vi "FindRequestByType.vi"(8 "ErrorIn":errorcluster={"status"=TRUE, "code"=6, "source"="Device disconnected"}, 11 "RequestType":T2=enum."Reset") -> (0 "ErrorOut":errorcluster={"status"=TRUE, "code"=6, "source"="Device disconnected"}, 3 "Request":T1={"Type"=enum."Reset", "Command"="", "Mode"={"Direction"=enum."TransmitOnly", "BytesToRead"=0}} {"Mode"."BytesToRead" min=1 max=4000000000 step=1})   [LabVIEW 2016]
doc: "Find Request cluster using its type. If the is no match during comparison with AvailableRequests, VI throws an error."
uses:
  RequestType.ctl
  Request.ctl
  FTDI/COMMode.ctl
  FTDI/COMDirection.ctl
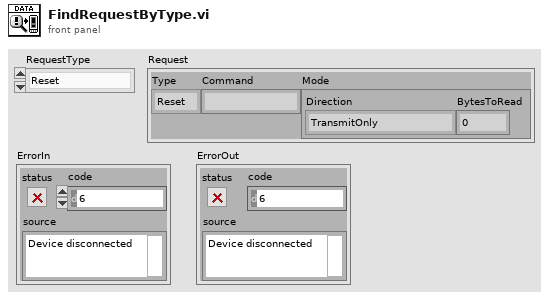
[diagram p1: front panel]
types:
  T1 = typedef "Request.ctl" = cluster{"Type":T2, "Command":string, "Mode":T3}
  T2 = typedef "RequestType.ctl" = enum16{"NONE", "Reset", "Hello", "GetPacketsNr", "GetMeasFreq", "GetPacket"}
  T3 = typedef "COMMode.ctl" = cluster{"Direction":T4, "BytesToRead":u32}
  T4 = typedef "COMDirection.ctl" = enum16{"CommandAndResponse", "ReceiveOnly", "TransmitOnly"}
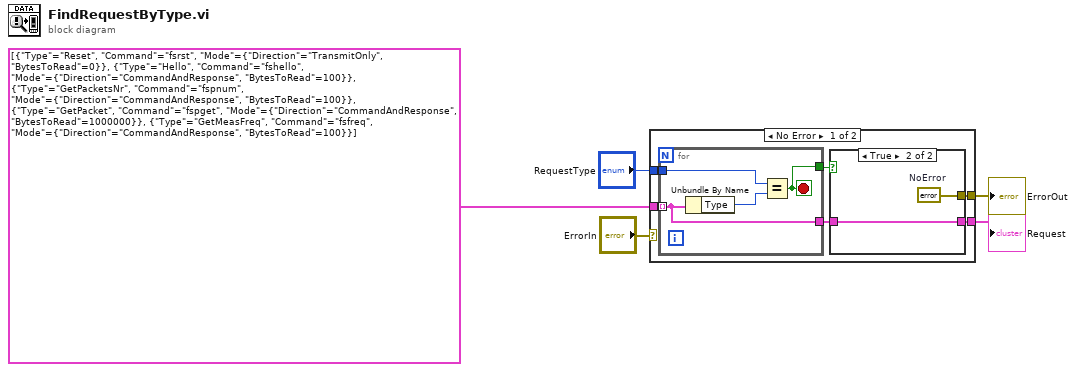
[diagram p0: block diagram]
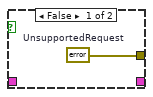
[diagram p2: hidden frame]
diagram:
  n1 = case shown="No Error" "ErrorIn" {
    selector: "ErrorIn" -> [_ w19]
    tunnel: "RequestType" -> [w11 _]
    tunnel: [w8 w19] -> w4
    tunnel: [w7 _] -> w3
    tunnel: T1[] [{"Type"=enum."Reset", "Command"="fsrst", "Mode"={"Direction"=enum."TransmitOnly", "BytesToRead"=0}}, {"Type"=enum."Hello", "Command"="fshello", "Mode"={"Direction"=enum."CommandAndResponse", "BytesToRead"=100}}, {"Type"=enum."GetPacketsNr", "Command"="fspnum", "Mode"={"Direction"=enum."CommandAndResponse", "BytesToRead"=100}}, {"Type"=enum."GetPacket", "Command"="fspget", "Mode"={"Direction"=enum."CommandAndResponse", "BytesToRead"=1000000}}, {"Type"=enum."GetMeasFreq", "Command"="fsfreq", "Mode"={"Direction"=enum."CommandAndResponse", "BytesToRead"=100}}] ("Requests") -> [w6 _]
    frame No Error {
      n2 = for {
        tunnel: w6 -> [w16] mode=indexing
        tunnel: w11 -> [w18]
        tunnel: [w16] -> w9
        tunnel: [w15] -> w10
        stop <- w15 stop-if-true
        n3 = Unbundle By Name(w16) -> ("Type"=w17:T2)
        n4 = Equal?(x=w18, y=w17) -> (x = y?=w15:bool)
      }
      n5 = case shown="True" w10 {
        tunnel: w9 -> [_ w13]
        tunnel: [w12 w14] -> w8
        tunnel: [_ w13] -> w7
        frame False {
          w12 = errorcluster {"status"=TRUE, "code"=6, "source"="Unsupported request"}  # UnsupportedRequest
        }
        frame True {
          w14 = errorcluster {"status"=FALSE, "code"=0, "source"=""}  # NoError
        }
      }
    }
    frame Error {
    }
  }
  "ErrorOut" <- w4
  "Request" <- w3
